vi "Configure InLimits.vi"(6 "In Limits Time (second) (1)":i32=1 min=1 max=60 step=1, 7 "Channel (0: Channel A)":u16(ring) items=["Channel A", "Channel B"], 8 "error in (no error)":errorcluster, 9 "In Limits (%FS) (0.01)":dbl=0.01 min=0.0 max=10.0 step=0.001, 11 "BH Druck PACE Series in":refnum<class "BH Druck PACE Series.lvclass">) -> (0 "error out":errorcluster, 3 "BH Druck PACE Series out":refnum<class "BH Druck PACE Series.lvclass">)   [LabVIEW 2022 SP3, in "BH Druck PACE Series.lvclass"]
uses:
  BH Druck PACE Series.lvclass
  BH Druck PACE Series.lvclass/BH Druck PACE Series.ctl
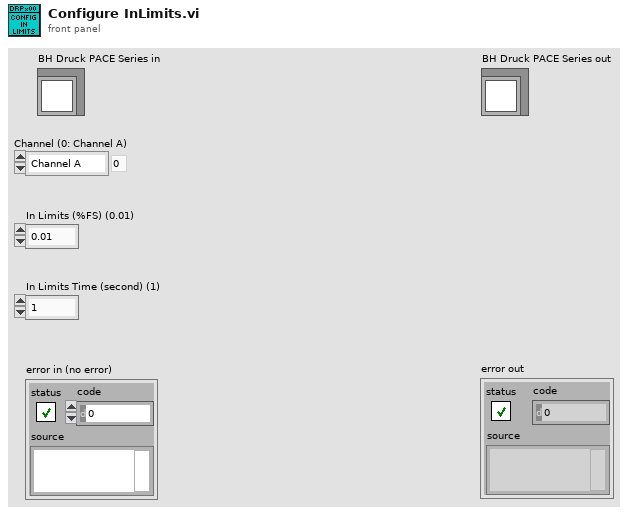
[diagram p1: front panel]
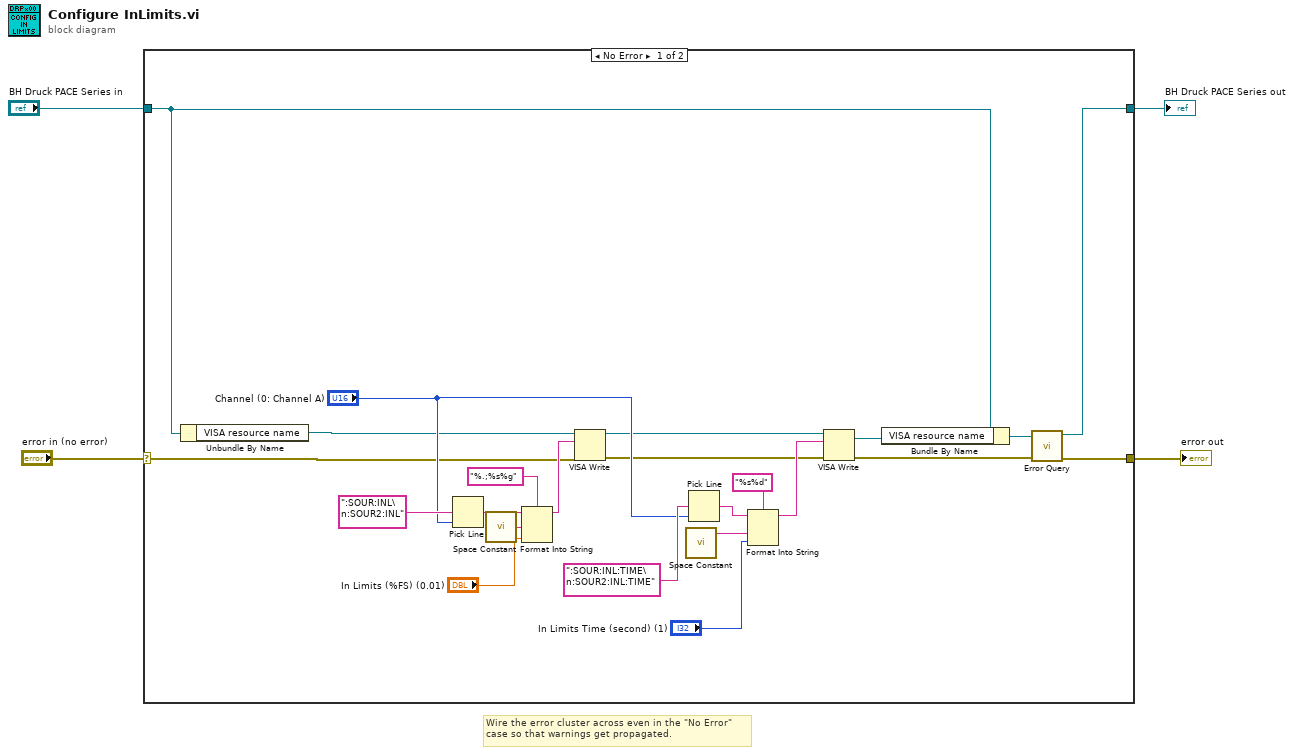
[diagram p0: block diagram]
diagram:
  # "Wire the error cluster across even in the \"No Error\"\ncase so that warnings get propagated."
  n1 = case shown="No Error" "error in (no error)" {
    selector: "error in (no error)" -> [w12 w29]
    tunnel: [w10 w29] -> w3
    tunnel: [w5 w28] -> w1
    tunnel: "BH Druck PACE Series in" -> [w8 w28]
    frame No Error {
      n2 = Unbundle By Name(w8) -> ("VISA resource name"=w9:refnum<visa-resource-name>)
      n3 = Pick Line(multi-line string=":SOUR:INL\n:SOUR2:INL", line index="Channel (0: Channel A)") -> (output string=w27:string)  [unwired: 1 in]
      n4 = call <vilib>:"Space Constant.vi"() -> ("String"=w24:string)
      n5 = Format Into String(format string="%.;%s%g", initial string=w27, w24, "In Limits (%FS) (0.01)") -> (resulting string=w26:string)  [unwired: 1 in, 1 out]
      n6 = VISA Write(VISA resource name=w9, write buffer=w26, error in (no error)=w12) -> (VISA resource name out=w15:refnum<visa-resource-name>, error out=w14:errorcluster)  [unwired: 1 out]
      n7 = call <vilib>:"Space Constant.vi"() -> ("String"=w18:string)
      n8 = Pick Line(multi-line string=":SOUR:INL:TIME\n:SOUR2:INL:TIME", line index="Channel (0: Channel A)") -> (output string=w21:string)  [unwired: 1 in]
      n9 = Format Into String(format string="%s%d", initial string=w21, w18, "In Limits Time (second) (1)") -> (resulting string=w20:string)  [unwired: 1 in, 1 out]
      n10 = VISA Write(VISA resource name=w15, write buffer=w20, error in (no error)=w14) -> (VISA resource name out=w7:refnum<visa-resource-name>, error out=w11:errorcluster)  [unwired: 1 out]
      n11 = Bundle By Name(cluster=w8, "VISA resource name"=w7) -> (w6:refnum<class "BH Druck PACE Series.lvclass">)
      n12 = call-dynamic "Error Query.vi"("error in (no error)"=w11, "BH Druck PACE Series in"=w6) -> ("error out"=w10:errorcluster, "BH Druck PACE Series out"=w5:refnum<class "BH Druck PACE Series.lvclass">)  [unwired: 8 in]
    }
    frame Error {
    }
  }
  "error out" <- w3
  "BH Druck PACE Series out" <- w1
